vi "Symmetrize (single).vi"(8 "error in (no error)":errorcluster, 11 "XY-data":cluster{"X-array":dbl[], "Y-array":dbl[]} {"Y-array" format="%.2p"; "X-array" format="%.2p"}) -> (0 "error out":errorcluster, 1 "Antisymmetric":cluster{"X-array":dbl[], dbl[]}, 2 "Symmetric":cluster{"X-array":dbl[], dbl[]}, 3 "XY-data out":cluster{"X-array":dbl[], "Y-array":dbl[]} {"Y-array" format="%.2p"; "X-array" format="%.2p"})   [LabVIEW 2019, in "xy_utilities.lvlib"]
doc: "Compute the Symmetric and Antisymmetric functions of <b>XY-data</b>\n\n<b>Symmetric</b>: f+ = (f(x) + f(-x))/2\n<b>Antisymmetric</b>: f- = (f(x) - f(-x))/2"
uses:
  xy_utilities.lvlib
  Sort (single).vi
  <userlib>/_OpenG.lib/array/array.llb/Sort Array__ogtk.vi
  <userlib>/_OpenG.lib/array/array.llb/Sort 1D Array (DBL)__ogtk.vi
  <userlib>/_OpenG.lib/array/array.llb/Reorder Array2__ogtk.vi
  <userlib>/_OpenG.lib/array/array.llb/Reorder 1D Array2 (DBL)__ogtk.vi
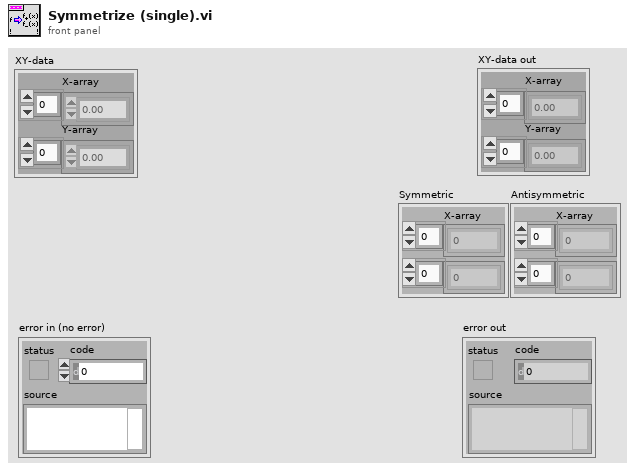
[diagram p1: front panel]
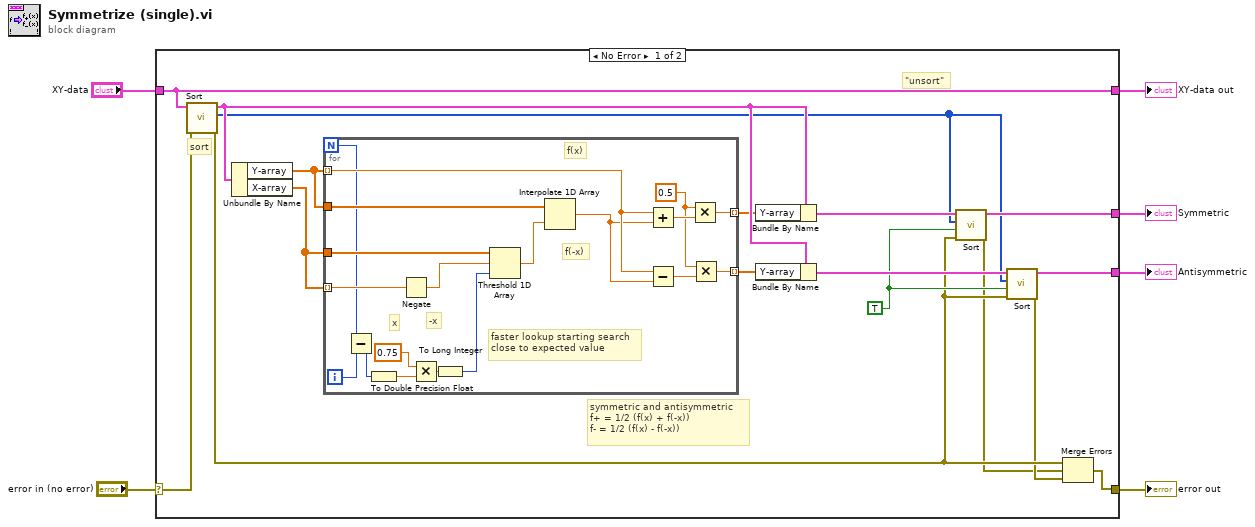
[diagram p0: block diagram]
diagram:
  n1 = case shown="No Error" "error in (no error)" {
    selector: "error in (no error)" -> [w23 w44]
    tunnel: [w12 w44] -> w5
    tunnel: "XY-data" -> [w7 w43]
    tunnel: [w7 w43] -> w3
    tunnel: [w18 _] -> w2
    tunnel: [w19 _] -> w1
    frame No Error {
      w17 = TRUE ("Use Sort Pointers (F)")
      # "sort"
      # "symmetric and antisymmetric\nf+ = 1/2 (f(x) + f(-x))\nf- = 1/2 (f(x) - f(-x))"
      # "\"unsort\""
      n2 = call-poly "Sort.vi"("error in (no error)"=w23, "XY-data"=w7) -> ("error out"=w15:errorcluster, "Sorted Pointers"=w16:i32[], "Sorted XY-data out"=w22:cluster{"X-array":dbl[], "Y-array":dbl[]})  [unwired: 7 in]
      n3 = Unbundle By Name(w22) -> ("Y-array"=w9:dbl[], "X-array"=w10:dbl[])
      n4 = for {
        N -> [w30]
        tunnel: [w33] -> w11 mode=indexing
        tunnel: [w32] -> w8 mode=indexing
        tunnel: w10 -> [w42] mode=indexing
        tunnel: w10 -> [w41]
        tunnel: w9 -> [w38]
        tunnel: w9 -> [w34] mode=indexing
        i -> [w29]
        w35 = 0.5 ("x")
        # "faster lookup starting search\nclose to expected value"
        # "f(x)"
        # "x"
        # "f(-x)"
        # "-x"
        n5 = Subtract(x=w30, y=w29) -> (x-y=w27:i32)
        n6 = To Double Precision Float(number=w27) -> (double precision float=w24:dbl)
        n7 = Negate(x=w42) -> (-x=w40:dbl)
        n8 = Multiply(x=0.75, y=w24) -> (x*y=w26:dbl)
        n9 = To Long Integer(number=w26) -> (32bit integer=w25:i32)
        n10 = Threshold 1D Array(1:w25, 2:w40, 3:w41) -> (0:w39:dbl)
        n11 = Interpolate 1D Array(1:w39, 2:w38) -> (0:w31:dbl)
        n12 = Add(x=w34, y=w31) -> (x+y=w37:dbl)
        n13 = Subtract(x=w34, y=w31) -> (x-y=w36:dbl)
        n14 = Multiply(x=w35, y=w37) -> (x*y=w33:dbl)
        n15 = Multiply(x=w35, y=w36) -> (x*y=w32:dbl)
      }
      n16 = Bundle By Name(cluster=w22, "Y-array"=w11) -> (w21:cluster{"X-array":dbl[], "Y-array":dbl[]})
      n17 = Bundle By Name(cluster=w22, "Y-array"=w8) -> (w20:cluster{"X-array":dbl[], "Y-array":dbl[]})
      n18 = call-poly "Sort.vi"("error in (no error)"=w15, "Use Sort Pointers (F)"=w17, "Sort Pointers"=w16, "XY-data"=w21) -> ("error out"=w13:errorcluster, "Sorted XY-data out"=w18:cluster{"X-array":dbl[], "Y-array":dbl[]})  [unwired: 5 in, 1 out]
      n19 = call-poly "Sort.vi"("error in (no error)"=w15, "Use Sort Pointers (F)"=w17, "Sort Pointers"=w16, "XY-data"=w20) -> ("error out"=w14:errorcluster, "Sorted XY-data out"=w19:cluster{"X-array":dbl[], "Y-array":dbl[]})  [unwired: 5 in, 1 out]
      n20 = Merge Errors(w15, w13, w14) -> (w12:errorcluster)
    }
    frame Error {
    }
  }
  "error out" <- w5
  "XY-data out" <- w3
  "Symmetric" <- w2
  "Antisymmetric" <- w1
